vi "Stop sampling.vi"(0 "RBD9103":T1, 5 "error in":errorcluster) -> (14 "RBD9103 out":T1, 19 "error out":errorcluster)   [LabVIEW 2018]
uses:
  RBD9103.ctl
  GenericDataEvent/GenericEvent.ctl
  Operation type.ctl
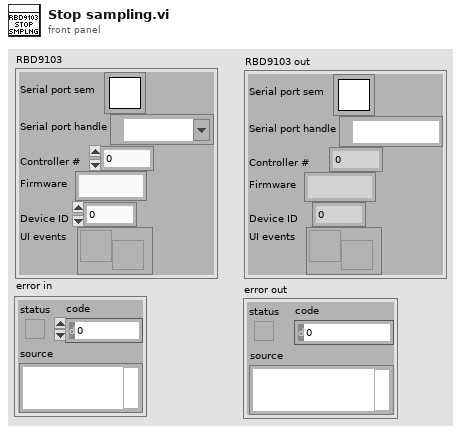
[diagram p1: front panel]
types:
  T1 = typedef "RBD9103.ctl" = cluster{"Serial port sem":T2, "Serial port handle":refnum<visa-resource-name>, "Controller #":u8, "Firmware":string, "Device ID":i32, "UI events":T3}
  T2 = typedef "Semaphore RefNum" = refnum<k1>
  T3 = typedef "GenericEvent.ctl" = refnum<user-event>
  T4 = typedef "Operation type.ctl" = enum16{"Write&Read", "Read only", "Write only", "Read only multiply"}
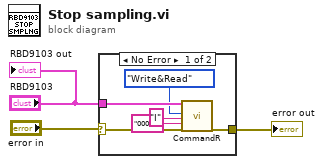
[diagram p0: block diagram]
diagram:
  n1 = case shown="No Error" "error in" {
    selector: "error in" -> [w5 w10]
    tunnel: [w8 w10] -> w1
    tunnel: "RBD9103" -> [w9 _]
    frame No Error {
      n2 = call "CommandR.vi"("RBD9103"=w9, "Operation"=Operation_type."Write&Read" ("Operation type"), "Command"="I", "Data"="0000" ("Command"), "error in"=w5) -> ("error out"=w8:errorcluster)  [unwired: 11 in, 3 out]
    }
    frame Error {
    }
  }
  "error out" <- w1
  "RBD9103 out" <- "RBD9103"
